vi "Simplify Malleable Instance Name.vi"(8 "error in (no error)":errorcluster, 10 "Fully Qualified Malleable VI Name":string, 11 "Fully Qualified Malleable Instance Name":string) -> (0 "error out":errorcluster, 3 "Simple Malleable Instance Name":string)   [LabVIEW 2020, in "Peek Window.lvlib" / "Malleable VI Type.lvclass"]
uses:
  Malleable VI Type.lvclass
  <vilib>/regexp/Match Regular Expression.xnode
  Malleable VI Type.lvclass/Malleable VI Type.ctl
  Peek Window.lvlib
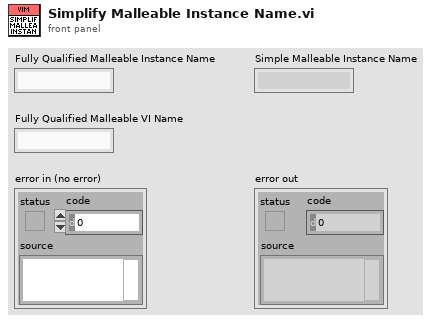
[diagram p1: front panel]
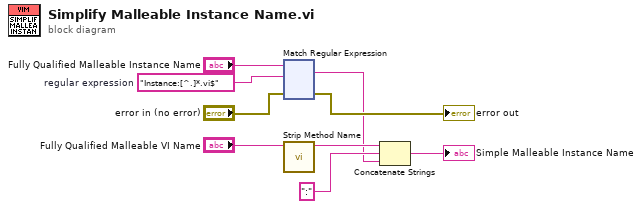
[diagram p0: block diagram]
diagram:
  w8 = "Instance:[^.]*.vi$"  # regular expression
  n1 = xnode "Match Regular Expression"("input string"="Fully Qualified Malleable Instance Name", "regular expression"=w8, "error in"="error in (no error)") -> ("whole match"=w1:string, "error out"=→"error out":errorcluster)  [unwired: 3 in, 3 out]
  n2 = call "Strip Method Name.vi"("Full Qualified Name in"="Fully Qualified Malleable VI Name") -> ("Plain Method Name out"=w4:string)  [unwired: 10 in]
  n3 = Concatenate Strings(w4, ":", w1) -> (→"Simple Malleable Instance Name":string)
